vi "testTransHexaPosCoorSys.vi"(8 "error in (no error)":errorcluster) -> (0 "error out":errorcluster)   [LabVIEW 2016]
doc: "Test the coordinate transformation between Zemax and optical coordinate systems for the hexapod position."
uses:
  SubSysAdap/SubSysAdap.lvclass
  <vilib>/addons/_JKI Toolkits/Caraya/classes/Test/Test.lvclass
  <vilib>/addons/_JKI Toolkits/Caraya/classes/Assert/Assert.lvclass
panel:
  in  "Configuration":T1={"Config Dir"=path "/home/ttsai/Documents/stash/ts_tcs_ofc/configData", "Rot Mirror FEA File Name"="rotMat_Bo_to_Chris_FEA_DOF.txt", "Rot Hexapod FEA File Name"="rotMat_hexapod.txt"}
  in  "SubSysAdap.lvclass":refnum<class "SubSysAdap.lvclass">
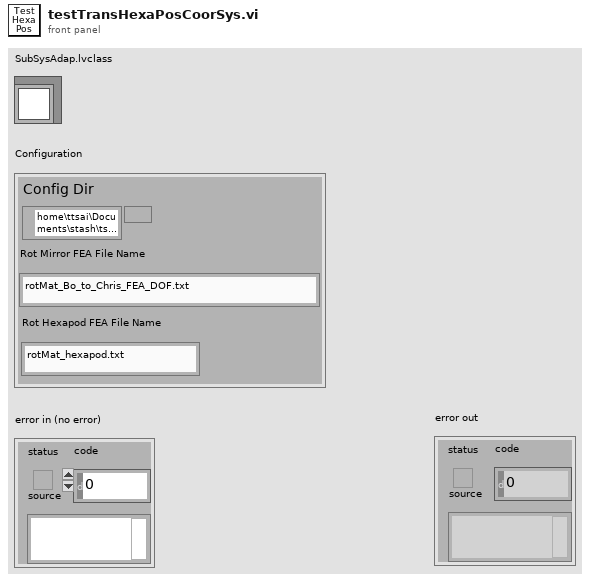
[diagram p1: front panel]
types:
  T1 = cluster{"Config Dir":path, "Rot Mirror FEA File Name":string, "Rot Hexapod FEA File Name":string}
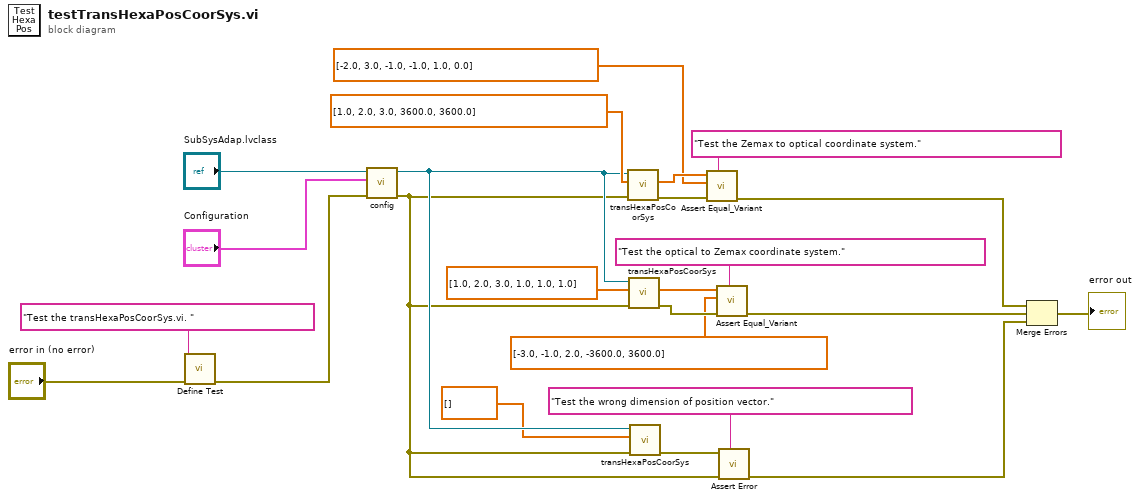
[diagram p0: block diagram]
diagram:
  n1 = call <vilib>:"Define Test.vi"("error in (no error)"="error in (no error)", "Label (VI Title)"="Test the transHexaPosCoorSys.vi. ") -> ("error out"=w19:errorcluster)  [unwired: 9 in]
  n2 = call "config.vi"("error in (no error)"=w19, "Configuration"="Configuration", "SubSysAdap in"="SubSysAdap.lvclass") -> ("error out"=w2:errorcluster, "SubSysAdap out"=w6:refnum<class "SubSysAdap.lvclass">)  [unwired: 7 in]
  n3 = call "transHexaPosCoorSys.vi"("error in (no error)"=w2, "Hex Pos"=dbl[] [1.0, 2.0, 3.0, 3600.0, 3600.0], "SubSysAdap in"=w6) -> ("error out"=w16:errorcluster, "Trans Hex Pos"=w14:dbl[])  [unwired: 6 in, 1 out]
  n4 = call "transHexaPosCoorSys.vi"("error in (no error)"=w2, "Hex Pos"=dbl[] [1.0, 2.0, 3.0, 1.0, 1.0, 1.0], "SubSysAdap in"=w6) -> ("error out"=w10:errorcluster, "Trans Hex Pos"=w11:dbl[])  [unwired: 6 in, 1 out]
  n5 = call "transHexaPosCoorSys.vi"("error in (no error)"=w2, "Hex Pos"=dbl[] [], "SubSysAdap in"=w6) -> ("error out"=w3:errorcluster)  [unwired: 6 in, 2 out]
  n6 = call <vilib>:"Assert Equal_Variant.vi"("Label"="Test the Zemax to optical coordinate system.", "error in (no error)"=w16, "Y"=dbl[] [-2.0, 3.0, -1.0, -1.0, 1.0, 0.0], "X"=w14) -> ("error out"=w15:errorcluster)  [unwired: 7 in]
  n7 = call <vilib>:"Assert Equal_Variant.vi"("Label"="Test the optical to Zemax coordinate system.", "error in (no error)"=w10, "Y"=dbl[] [-3.0, -1.0, 2.0, -3600.0, 3600.0], "X"=w11) -> ("error out"=w7:errorcluster)  [unwired: 7 in]
  n8 = call <vilib>:"Assert Error.vi"("Label"="Test the wrong dimension of position vector.", "error in (no error)"=w2, "Error?"=w3) -> ("error out"=w5:errorcluster)  [unwired: 8 in]
  n9 = Merge Errors(w15, w7, w5) -> (→"error out":errorcluster)
